vi "探测器列表-删除设备.vi"(7 "table名-探测器列表":string, 8 "error in (no error)":errorcluster, 10 "网络地址":string, 11 "数据库引用":T1) -> (0 "error out":errorcluster, 3 "connection reference out":T1)   [LabVIEW 2017]
uses:
  <vilib>/addons/database/Connection.llb/Conn ObjectReference.ctl
  <vilib>/addons/database/NI_Database_API.lvlib
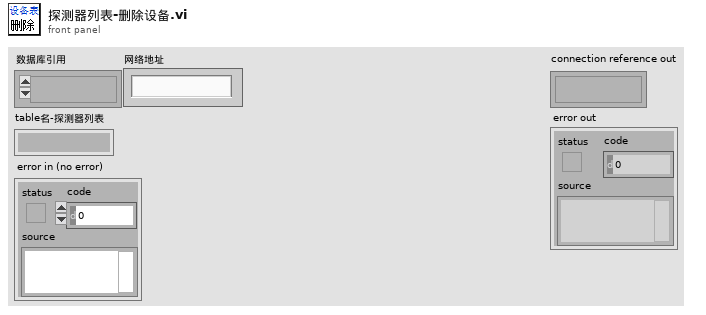
[diagram p1: front panel]
types:
  T1 = typedef "NI_Database_API.lvlib/Conn ObjectReference.ctl" = refnum<k1>
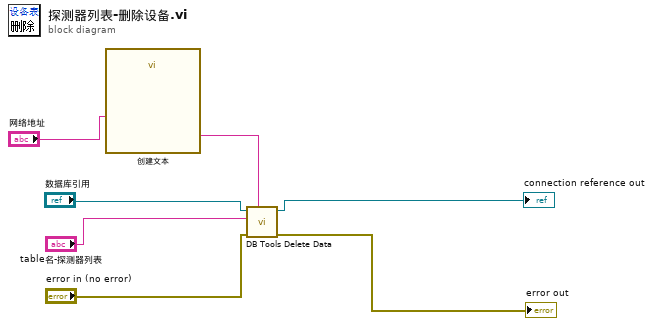
[diagram p0: block diagram]
diagram:
  n1 = call "创建文本"("网络地址"="网络地址") -> ("Result"=w1:string)  [unwired: 13 in, 1 out]
  n2 = call <vilib>:"DB Tools Delete Data.vi"("condition"=w1, "error in (no error)"="error in (no error)", "table"="table名-探测器列表", "connection reference"="数据库引用") -> ("error out"=→"error out":errorcluster, "connection reference out"=→"connection reference out":T1)  [unwired: 6 in]
